vi "Generate Report.vi"(8 "error in (no error)":errorcluster, 10 "Generate Report":bool, 11 "Test Application Controller in":refnum<class "Test Application Controller.lvclass">) -> (0 "error out":errorcluster, 3 "Test Application Controller out":refnum<class "Test Application Controller.lvclass">)   [LabVIEW 2017, in "Test Application Controller.lvlib" / "Test Application Controller.lvclass"]
uses:
  Test Application Controller.lvclass
  Test Application Controller.lvclass/Test Application Controller.ctl
  <vilib>/ActorFramework/Message Enqueuer/Message Enqueuer.lvclass/Message Enqueuer.ctl
  <vilib>/ActorFramework/Message Enqueuer/Enqueue.vi
  Test/Test Messages/Generate Report Msg/Generate Report Msg.lvclass
  C:/Program Files (x86)/National Instruments/LabVIEW 2017/vi.lib/ActorFramework/Message/Message.lvclass
  <vilib>/ActorFramework/Message Priority Queue/Priority Enqueue.vi
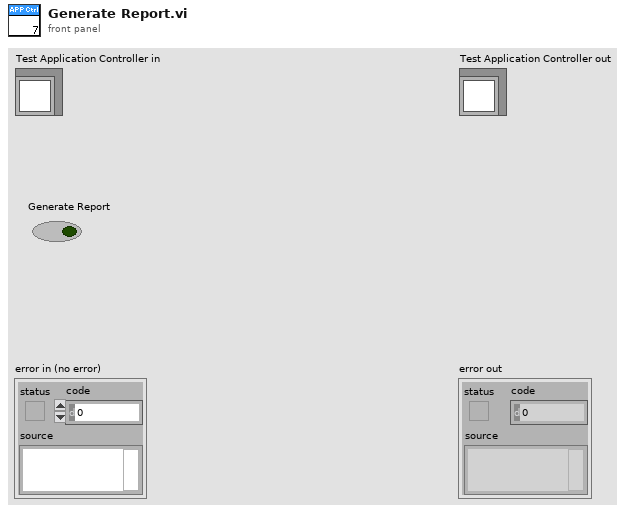
[diagram p1: front panel]
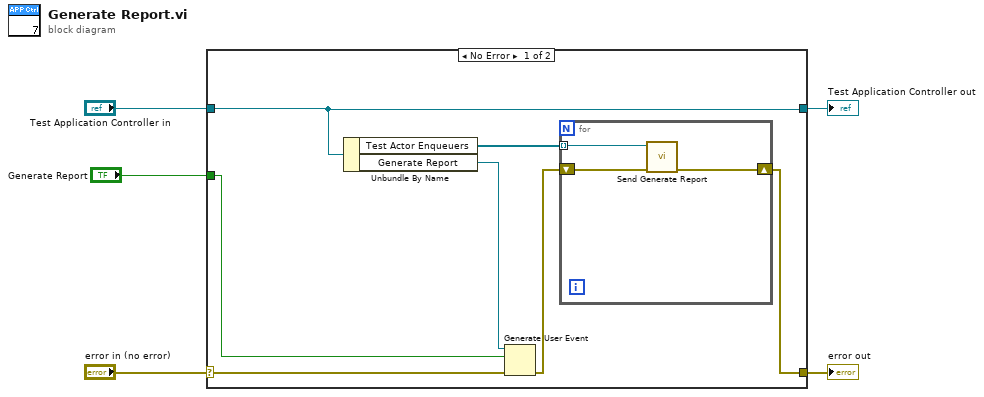
[diagram p0: block diagram]
diagram:
  n1 = case shown="No Error" "error in (no error)" {
    selector: "error in (no error)" -> [w10 w17]
    tunnel: [w6 w17] -> w4
    tunnel: [w9 w16] -> w2
    tunnel: "Test Application Controller in" -> [w9 w16]
    tunnel: "Generate Report" -> [w11 _]
    frame No Error {
      n2 = Unbundle By Name(w9) -> ("Test Actor Enqueuers"=w8:refnum<class "Message Enqueuer.lvclass">[], "Generate Report"=w12:refnum<user-event>)
      n3 = Generate User Event(user event=w12, event data cluster=w11, error in=w10) -> (error out=w7:errorcluster)  [unwired: 1 in, 1 out]
      n4 = for {
        tunnel: w8 -> [w15] mode=indexing
        shift-right: [w13] -> w6
        shift-left: w7 -> [w14]
        n5 = call "Send Generate Report.vi"("error in (no error)"=w14, "Message Enqueuer"=w15) -> ("error out"=w13:errorcluster)  [unwired: 8 in, 1 out]
      }
    }
    frame Error {
    }
  }
  "error out" <- w4
  "Test Application Controller out" <- w2
